vi "Default Instrument Setup.vi"(8 "error in (no error)":errorcluster, 11 "VISA resource name":refnum<visa-resource-name>) -> (0 "error out":errorcluster, 3 "VISA resource name out":refnum<visa-resource-name>)   [LabVIEW 2014, in "Agilent 34401.lvlib"]
doc: "This Utility VI sends a default command string to the instrument whenever a new VISA session is opened, or the instrument is reset. This VI is intended to be used as a subVI for the <B>Initialize</B> and <B>Reset</B> VI's. Altering this VI could cause these two VI's to operate incorrectly."
uses:
  <instrlib>/Agilent 34401/Agilent 34401.lvlib
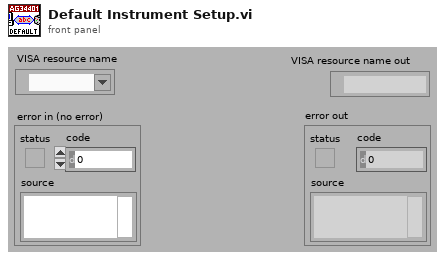
[diagram p1: front panel]
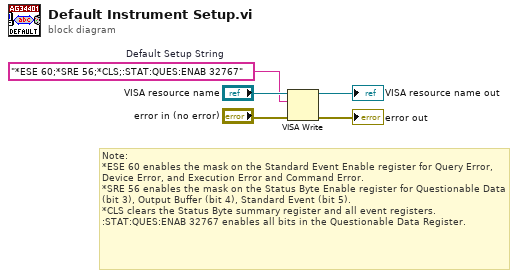
[diagram p0: block diagram]
diagram:
  w1 = "*ESE 60;*SRE 56;*CLS;:STAT:QUES:ENAB 32767"  # Default Setup String
  # "Note:\n*ESE 60 enables the mask on the Standard Event Enable register for Query Error, Device Error, and Execution Error and Command Error.\n*SRE 56 enables the mask on the Status Byte Enable register for Questionable Data (bit 3), Output Buffer (bit 4), Standard Event (bit 5).\n*CLS clears the Status Byte summary register and all event registers.\n:STAT:QUES:ENAB 32767 enables all bits in the Questionable Data Register."
  n1 = VISA Write(VISA resource name="VISA resource name", write buffer=w1, error in (no error)="error in (no error)") -> (VISA resource name out=→"VISA resource name out":refnum<visa-resource-name>, error out=→"error out":errorcluster)  [unwired: 1 out]
